vi "WS1050_PIC_RFFE_2K_Cycles.vi"(8 "error in (no error)":errorcluster, 9 "Initialize":bool, 10 "Number of Cycles":i32=50, 11 "VISA resource name 2":refnum<visa-resource-name>) -> (0 "error out":errorcluster, 2 "No of Cycles Completed":i32, 3 "VISA resource name out":refnum<visa-resource-name>)   [LabVIEW 2017]
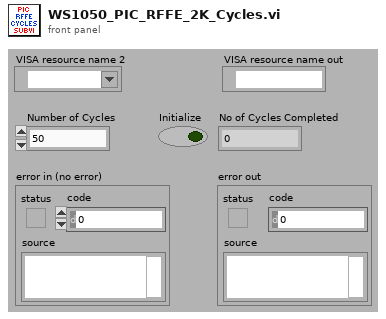
[diagram p1: front panel]
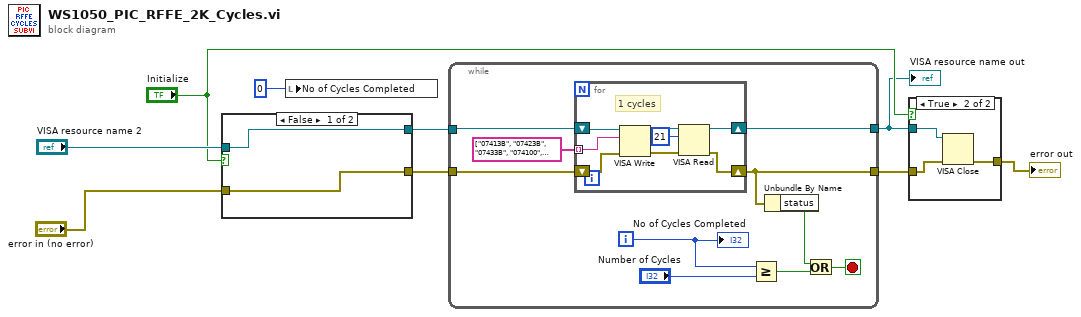
[diagram p0: block diagram]
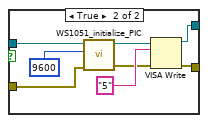
[diagram p3: hidden frame]
diagram:
  n1 = case shown="False" "Initialize" {
    tunnel: "error in (no error)" -> [w10 w18]
    tunnel: [w10 w12] -> w8
    tunnel: "VISA resource name 2" -> [w11 w17]
    tunnel: [w11 w13] -> w7
    frame False {
    }
    frame True {
      n2 = call "WS1051_initialize_PIC.vi"("error in (no error)"=w18, "baud rate"=u32 9600, "Select Com Port"=w17) -> ("error out"=w15:errorcluster, "VISA resource name out"=w14:refnum<visa-resource-name>)  [unwired: 7 in]
      n3 = VISA Write(VISA resource name=w14, write buffer="5", error in (no error)=w15) -> (VISA resource name out=w13:refnum<visa-resource-name>, error out=w12:errorcluster)  [unwired: 1 out]
    }
  }
  n4 = local write "No of Cycles Completed"(0 ("No of Cycles Completed")) -> ()
  n5 = while {
    tunnel: w8 -> [w29]
    tunnel: w7 -> [w28]
    tunnel: [w27] -> w1
    tunnel: [w26] -> w3
    i -> [w25]
    stop <- w23 stop-if-true
    n6 = for {
      tunnel: string[] ["07413B", "07423B", "07433B", "074100", "074200", "074300"] -> [w37] mode=indexing
      shift-right: [w33] -> w26
      shift-left: w29 -> [w35]
      shift-right: [w34] -> w27
      shift-left: w28 -> [w36]
      # "1 cycles"
      n7 = VISA Write(VISA resource name=w36, write buffer=w37, error in (no error)=w35) -> (VISA resource name out=w31:refnum<visa-resource-name>, error out=w32:errorcluster)  [unwired: 1 out]
      n8 = VISA Read(VISA resource name=w31, byte count=u32 21, error in (no error)=w32) -> (VISA resource name out=w34:refnum<visa-resource-name>, error out=w33:errorcluster)  [unwired: 2 out]
    }
    n9 = Greater Or Equal?(x=w25, y="Number of Cycles") -> (x >= y?=w21:bool)
    n10 = Unbundle By Name(w26) -> ("status"=w22:bool)
    n11 = Or(x=w22, y=w21) -> (x .or. y?=w23:bool)
    "No of Cycles Completed" <- w25
  }
  "VISA resource name out" <- w1
  n12 = case shown="True" "Initialize" {
    tunnel: w1 -> [_ w41]
    tunnel: w3 -> [w38 w40]
    tunnel: [w38 w39] -> w2
    frame False {
    }
    frame True {
      n13 = VISA Close(VISA resource name=w41, error in (no error)=w40) -> (error out=w39:errorcluster)
    }
  }
  "error out" <- w2
